vi "Suport SingleChannel PI Controller.vi"(0 "input data":fxp<+/-,21,6>, 5 "Integral Coefficient b[k]":fxp<+/-,18,1>, 7 "Integral Coefficient a[k]":fxp<+/-,18,2>, 9 "input valid":bool, 12 "reset":bool) -> (4 "output data":fxp<+/-,20,5> format="%.31g", 10 "output valid":bool, 14 "ready for input":bool)   [LabVIEW 2011, in "Filter VIs.lvlib"]
doc: "----------------------\n\nThis filter is configured as follows:\n\n<b>Filter Configuration</b>\nType: Single Rate\nStructure: IIR Cascaded Second-Order Sections Form II Transposed\n\n<b>Input Data Type</b>\nType: fixed-point <±,20,5> [-1.600000E+1,1.599997E+1]:3.051758E-5\n\n<b>Output Data Type</b>\nType: fixed-point <±,20,5> [-1.600000E+1,1.599997E+1]:3.051758E-5\nRounding mode: Round-Half-Even\nOverflow mode: Wrap\n\n<b>Implementation</b>\nNumber of channels: 1\nMaximum input sampling rate per channel @ 40MHz: 13.333MHz\nGain processing: On Target\nMethod: Multiply-Accumulate\n\n<b>Execution Mode</b>\nInside single-cycle Timed Loop\nThroughput: 3 cycles/sample\n\n<b>Estimated Resources</b>\n2 24x32 multiplier"
uses:
  Filter VIs.lvlib
  <vilib>/rvi/FXPMathLib/FxpMul/XNode/nifxpmath_Multiplier.xnode
  <vilib>/rvi/FXPMathLib/basic elements/FxpDiscreteDelay/XNode/nifxpmath_DiscreteDelay.xnode
  <vilib>/rvi/FXPMathLib/sim/FxpSim.dll
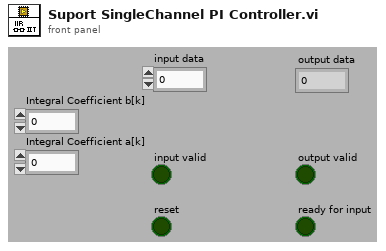
[diagram p1: front panel]
types:
  T1 = cluster{"update  v?":bool, "write s1?":bool, "init?":bool}
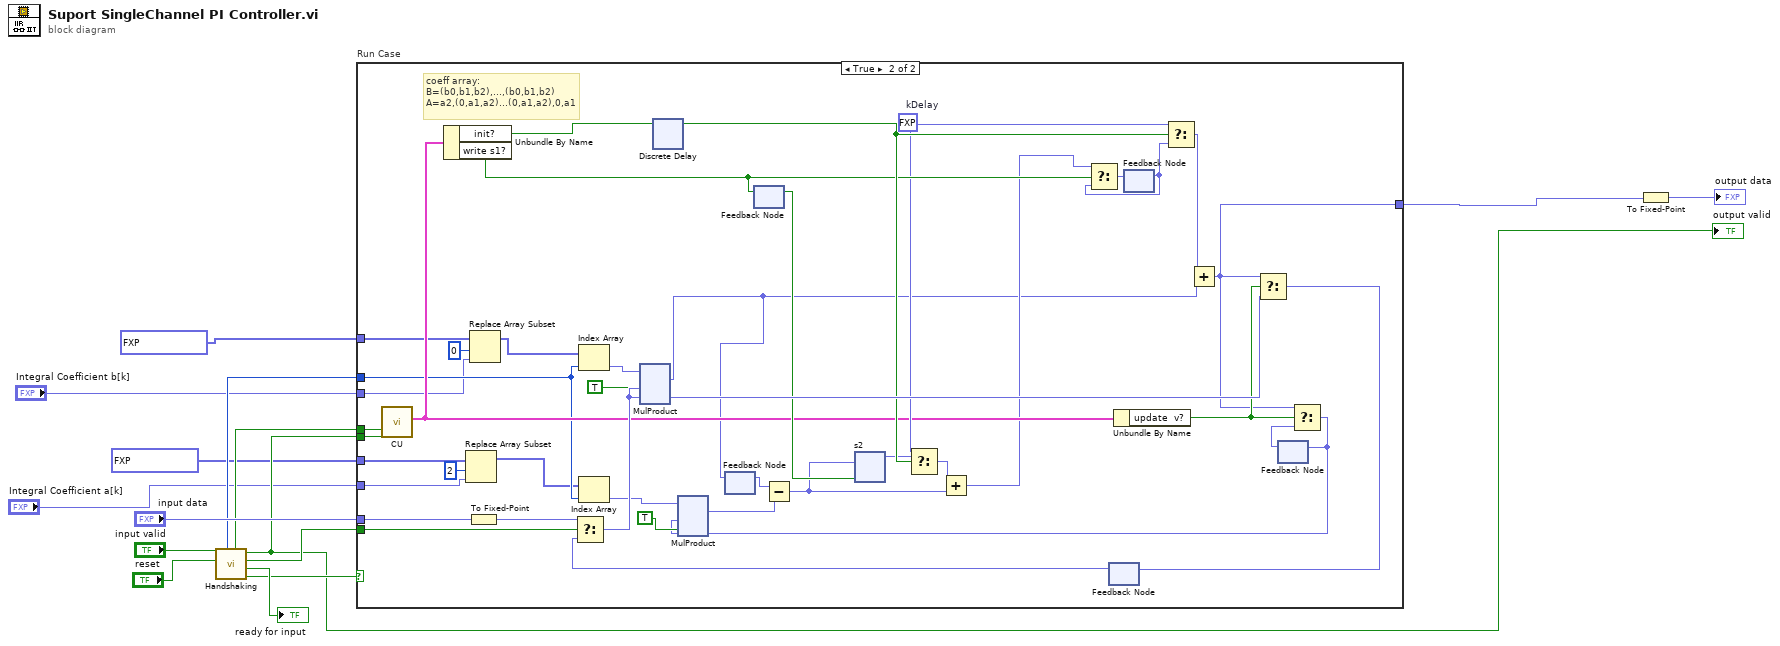
[diagram p0: block diagram]
diagram:
  n1 = call "Handshaking"("reset"="reset", "input valid"="input valid") -> ("run?"=w12:bool, "ready for input"=→"ready for input":bool, "load"=w8:bool, "output valid"=w5:bool, "reset for cu"=w11:bool, "idx"=w9:i16)  [unwired: 4 out]
  "output valid" <- w5
  n2 = case "Run Case" shown="True" w12 {
    tunnel: "input data" -> [_ w24]
    tunnel: w5 -> [_ w48]
    tunnel: w8 -> [_ w25]
    tunnel: w11 -> [_ w47]
    tunnel: w9 -> [_ w27]
    tunnel: [_ w28] -> w6
    tunnel: fxp<+/-,18,1>[] [0.5, 0.0, 0.0] ("coeff_b") -> [_ w23]
    tunnel: "Integral Coefficient b[k]" -> [_ w21]
    tunnel: fxp<+/-,18,2>[] [0.0, 0.0, -0.5] ("coeff_a") -> [_ w19]
    tunnel: "Integral Coefficient a[k]" -> [_ w17]
    frame False {
    }
    frame True {
      w34 = fxp<+/-,32,6> 0.0  # kDelay
      # "coeff array:\nB=(b0,b1,b2),...,(b0,b1,b2)\nA=a2,(0,a1,a2)...(0,a1,a2),0,a1"
      n3 = call "CU"("output valid"=w48, "global reset"=w47) -> ("Control signal"=w33:T1)  [unwired: 9 out]
      n4 = Unbundle By Name(w33) -> ("init?"=w46:bool, "write s1?"=w35:bool)
      n5 = Replace Array Subset(array=w19, new element=w17, index=2) -> (w16:fxp<+/-,18,2>[])
      n6 = To Fixed-Point ("toMultiplicand")(number=w24) -> (fixed-point=w54:fxp<+/-,32,6>)  [unwired: 1 out]
      n7 = Replace Array Subset(array=w23, new element=w21, index=0) -> (w20:fxp<+/-,18,1>[])
      n8 = Index Array(array=w20, index=w27) -> (element=w53:fxp<+/-,18,1>)
      n9 = Index Array(array=w16, index=w27) -> (element=w36:fxp<+/-,18,2>)
      n10 = xnode ("Discrete Delay")("D"=w46) -> ("Q"=w44:bool)
      n11 = feedback #1() -> (w40:fxp<+/-,32,6>)  [unwired: 1 out]
      n12 = feedback-in #2(w35) -> ()
      n13 = feedback #2() -> (w42:bool)  [unwired: 1 out]
      n14 = feedback #3() -> (w50:fxp<+/-,32,6>)  [unwired: 1 out]
      n15 = Select(t=w54, s=w25, f=w50) -> (s? t:f=w52:fxp<+/-,32,6>)
      n16 = xnode "MulProduct"("x"=w53, "y"=w52, "input valid"=TRUE) -> ("x*y"=w26:fxp<+/-,32,6>)  [unwired: 1 in, 2 out]
      n17 = feedback-in #1(w26) -> ()
      n18 = Unbundle By Name(w33) -> ("update  v?"=w49:bool)
      n19 = feedback #4() -> (w38:fxp<+/-,32,6>)  [unwired: 1 out]
      n20 = Select(t=w34, s=w44, f=w38) -> (s? t:f=w51:fxp<+/-,32,6>)
      n21 = Add ("AddSum")(x=w51, y=w26) -> (x+y=w28:fxp<+/-,32,6>)
      n22 = Select(t=w28, s=w49, f=w52) -> (s? t:f=w30:fxp<+/-,32,6>)
      n23 = feedback-in #3(w30) -> ()
      n24 = feedback #5() -> (w41:fxp<+/-,32,6>)  [unwired: 1 out]
      n25 = Select(t=w28, s=w49, f=w41) -> (s? t:f=w29:fxp<+/-,32,6>)
      n26 = xnode "MulProduct"("x"=w36, "y"=w29, "input valid"=TRUE) -> ("x*y"=w55:fxp<+/-,32,6>)  [unwired: 1 in, 2 out]
      n27 = Subtract ("SubSum")(x=w40, y=w55) -> (x-y=w31:fxp<+/-,32,6>)
      n28 = xnode ("s2")("D"=w31, "enable"=w42) -> ("Q"=w43:fxp<+/-,32,6>)
      n29 = Select(t=w34, s=w44, f=w43) -> (s? t:f=w45:fxp<+/-,32,6>)
      n30 = Add ("AddSum")(x=w45, y=w31) -> (x+y=w32:fxp<+/-,32,6>)
      n31 = Select(t=w32, s=w35, f=w38) -> (s? t:f=w39:fxp<+/-,32,6>)
      n32 = feedback-in #4(w39) -> ()
      n33 = feedback-in #5(w29) -> ()
    }
  }
  n34 = To Fixed-Point ("toOutput")(number=w6) -> (fixed-point=→"output data":fxp<+/-,20,5>)  [unwired: 1 out]
